vi "Append Image to Report.vi"   [LabVIEW 2017, in "NI_report.lvclass"]
doc: "For an HTML report, the VI embeds a link to an image into the report. (Windows) For a standard report, the VI appends the image from a file. Standard reports support .bmp, .gif, .wmf, .emf, and .jpg image files. \n\nYou can wire either a path to the image or a string that contains the image URL to this polymorphic VI. Wire data to the <B>path or URL of image</B> input to determine the polymorphic instance to use or manually select the instance."
uses:
  <vilib>/Utility/NIReport.llb/NI_report.lvclass
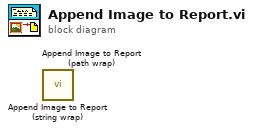
[diagram p0: block diagram]
diagram:
  n1 = call <vilib>:"Append Image to Report (string wrap).vi"() -> ()  [unwired: 12 in, 4 out]
  n2 = call <vilib>:"Append Image to Report (path wrap).vi"() -> ()  [unwired: 12 in, 4 out]
